vi "TCSPD.VI"() -> ()   [LabVIEW 2018, in "Shared_160.lvlib"]
uses:
  Shared_160.lvlib
  Global_Telescopio.vi
  tele.llb/TCSPD Globals.vi
panel:
  in  "OFF AUX":bool
  in  "EMERGÊNCIA":bool
  in  "Telescópio":bool
  out "Instrumento da Missão":string
  in  "Tabela Proteção":string[][](table)=[["Coude", "281.52", " 11.53", "S", "S", "0.462", "23.1", "23.1"], ["Cassegrain", "281.52", " 11.53", "S", "S", "0.462", "23.1", "23.1"], ["Eucalyptus", "281.52", " 11.53", "S", "S", "0.462", "23.1", "23.1"], ["Cam 1", "281.52", " 11.53", "S", "S", "0.462", "23.1", "23.1"], ["Cam 2", "281.52", " 11.53", "S", "S", "0.462", "23.1", "23.1"], ["Cam IV", "281.52", " 11.53", "S", "S", "0.462", "23.1", "23.1"], ["Polarimetro", "281.52", " 11.53", "S", "S", "0.462", "23.1", "23.1"], ["Fortrap", "281.52", " 11.53", "S", "S", "0.462", "23.1", "23.1"]]
  in  "CorrecaoMin":dbl=0.1
  out "Instrumento":u16(ring) items=["Coude A+", "Coude B+", "ECass+", "Eucalyptus+", "Cam 1+", "Cam 2*", "Cam4 + IV*", "Polarimetro*", "Fortrap*", "Cam1 RF*", "Coude C+", "MUSICOS*", "+Já testado", "* nao config", "cam 1 s/rf", "cam1srf/luca+focali", "Coude A/luca", "ECass/luca", "Cam1+rf+luca", "MUSICOS+Luca", "Camiv+Luca", "Cam2+Luca", "Cam1+rf+luca+Ixon", "Cam1+rf+luca+Ikon", "CoudeTeste", "*cam1srf/luca+focali", "cam1 + esp_focal", "SPARC4"]
  in  "tel_sts1":bool[](array[boolean])=[TRUE, TRUE, TRUE, TRUE, FALSE, FALSE, TRUE]
  out "String 4":string
  out "String 2":string
  out "String 3":string
  out "String":string
  in  "Boolean":bool
  out "Data Socket Test":dbl
  out "URL Temperatura":string
  in  "Reset_uC":bool
  in  "Password":string
  out "error out":errorcluster
  in  "sair":bool
  in  "ENGENHARIA":bool
  in  "SETUP":bool
  in  "Web Server:TCP/IP Access List":string[](array[string])=["c+*", "+observacao.vi"]
  # "TCSPD"
  # "TELESCOPE CONTROL SYSTEM\nPICO DOS DIAS OBSERVATORY"
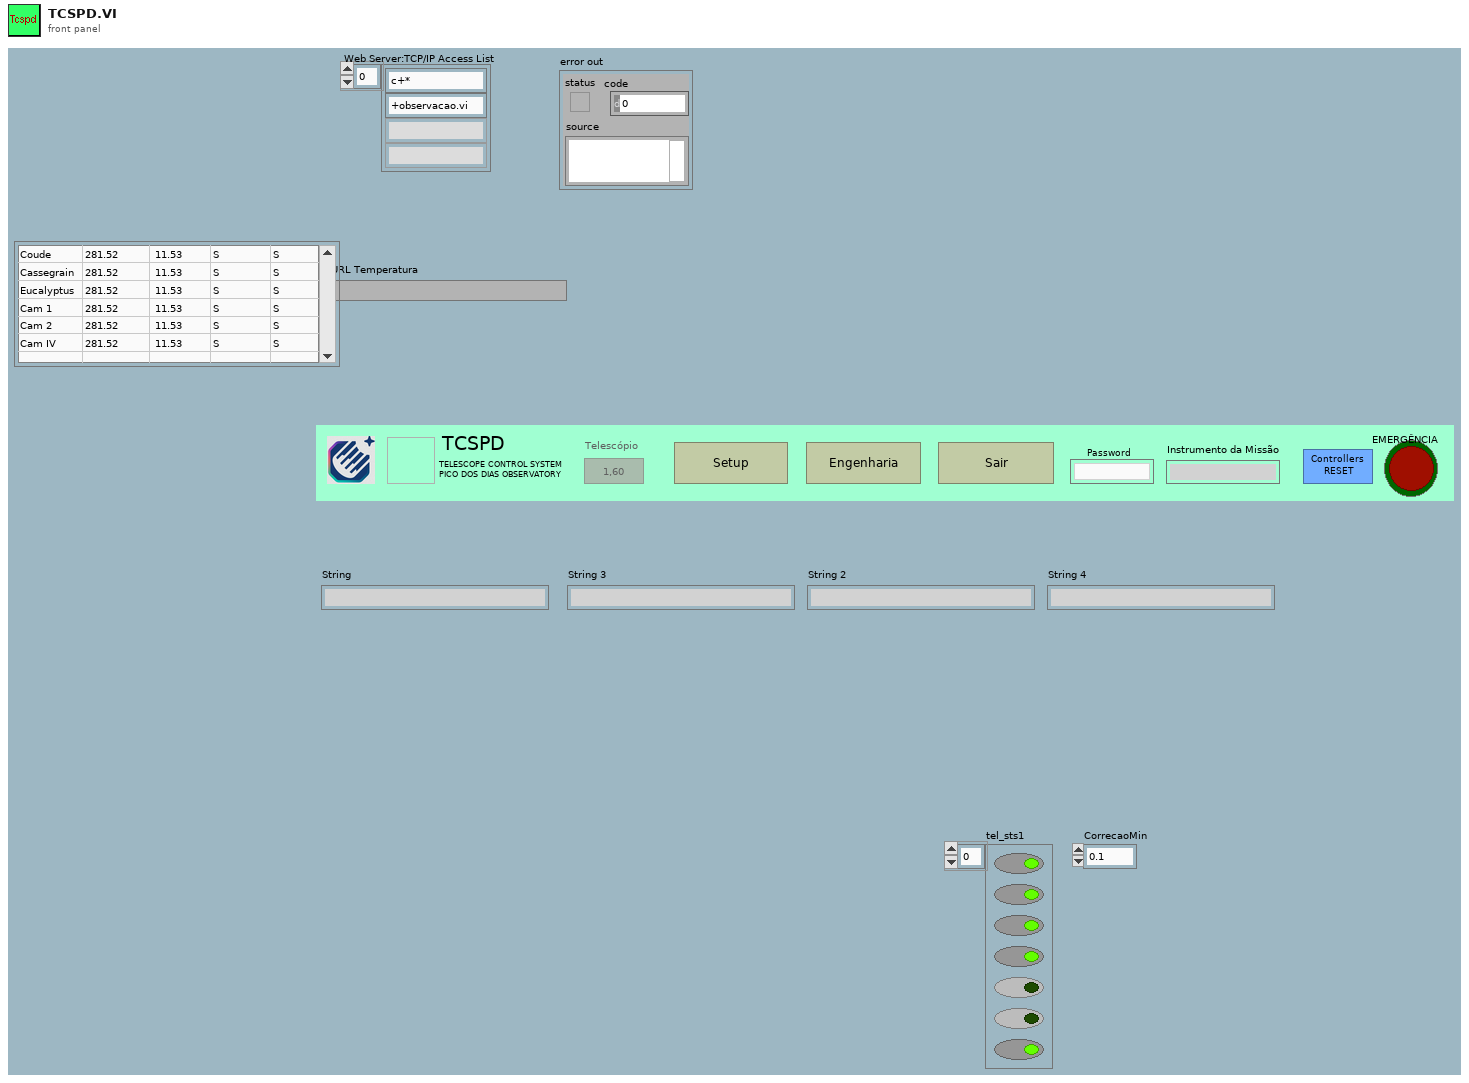
[diagram p1: front panel]
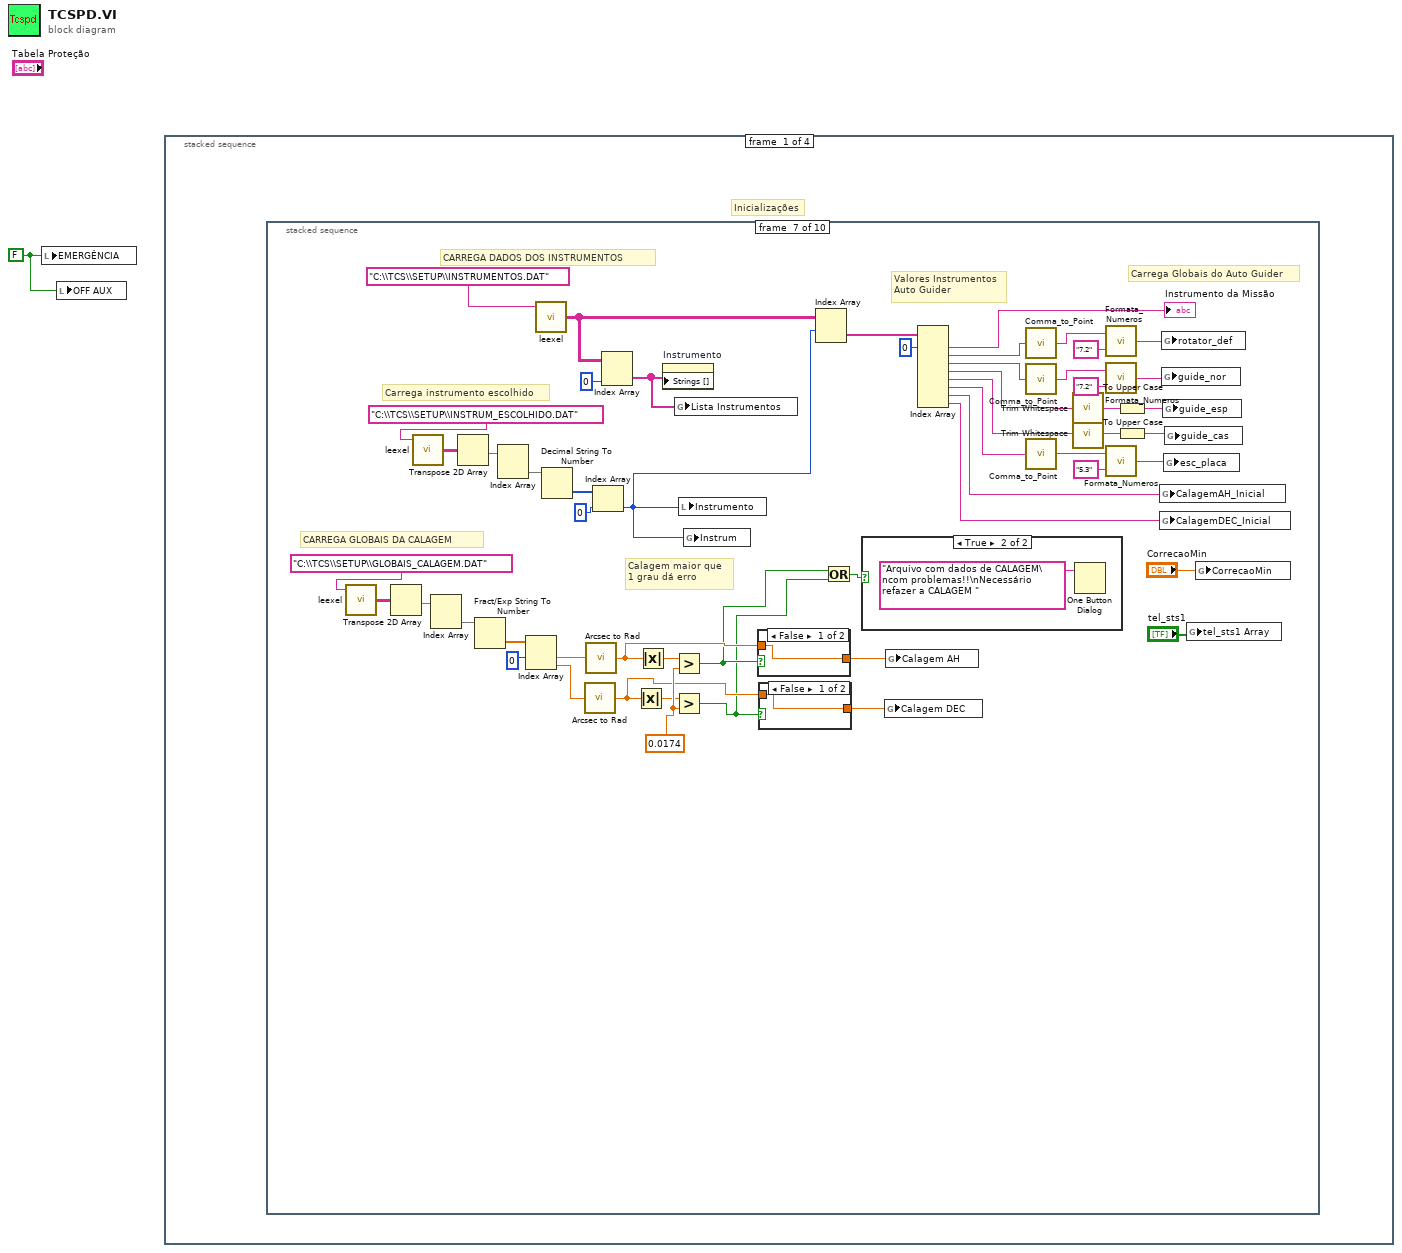
[diagram p0: block diagram]
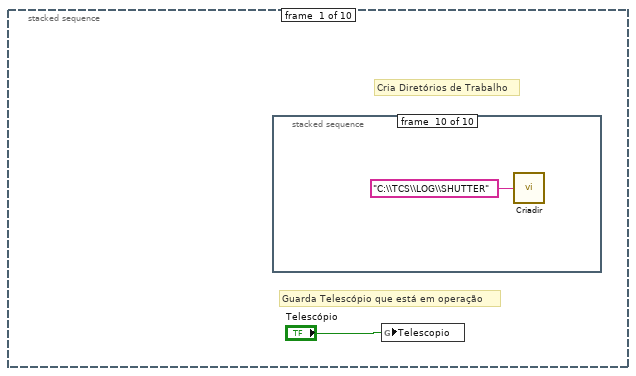
[diagram p2: hidden frame]
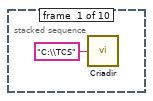
[diagram p3: hidden frame]
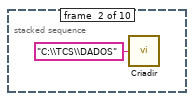
[diagram p4: hidden frame]
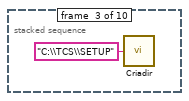
[diagram p5: hidden frame]
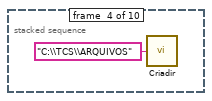
[diagram p6: hidden frame]
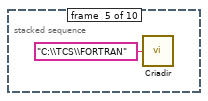
[diagram p7: hidden frame]
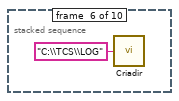
[diagram p8: hidden frame]
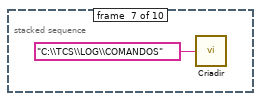
[diagram p9: hidden frame]
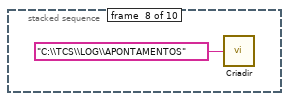
[diagram p10: hidden frame]
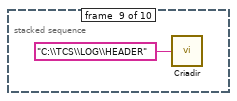
[diagram p11: hidden frame]
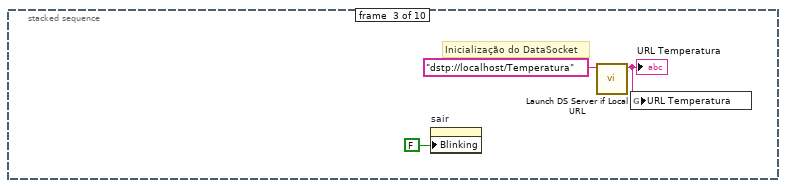
[diagram p13: hidden frame]
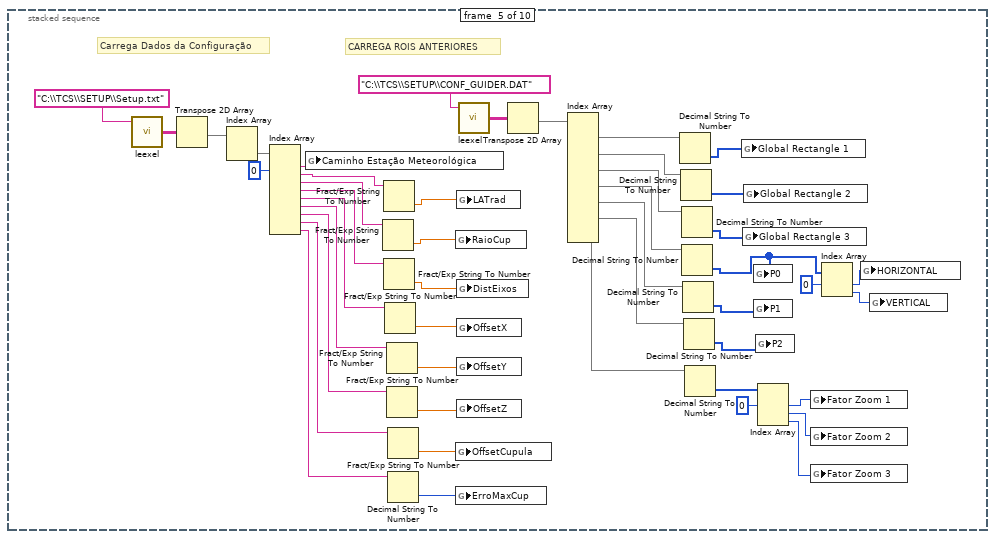
[diagram p15: hidden frame]
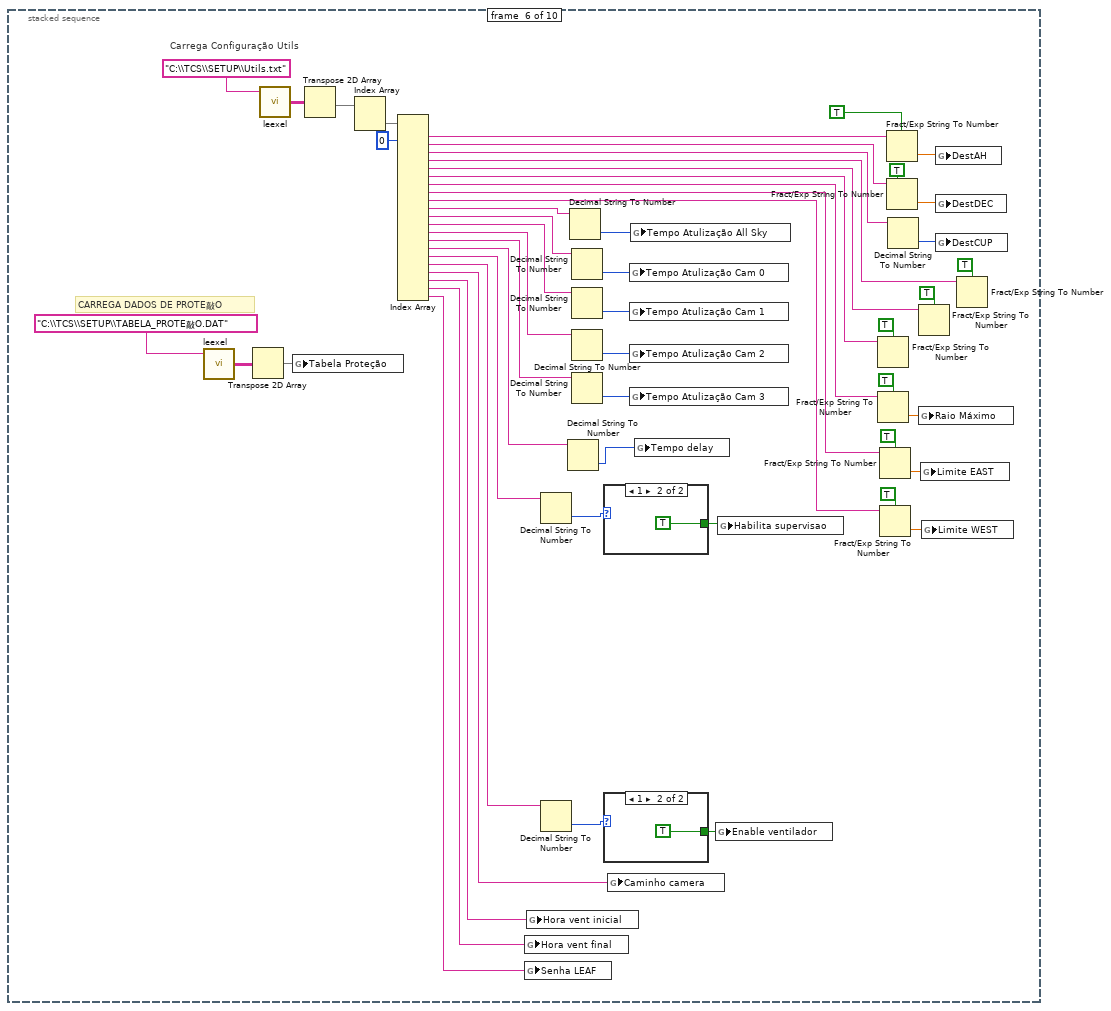
[diagram p16: hidden frame]
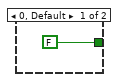
[diagram p17: hidden frame]
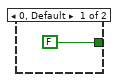
[diagram p18: hidden frame]
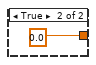
[diagram p20: hidden frame]
diagram:
  w1 = FALSE ("OFF")
  n1 = local write "EMERGÊNCIA"(w1) -> ()
  n2 = local write "OFF AUX"(w1) -> ()
  n3 = stacked-sequence {
    frame #0 {
      # "Inicializações"
      n4 = stacked-sequence {
        frame #0 {
          # "Guarda Telescópio que está em operação"
          # "Cria Diretórios de Trabalho"
          n5 = stacked-sequence {
            frame #0 {
              n6 = call "Criadir.vi"("SOMENTE DIRETORIO"="C:\\TCS") -> ()  [unwired: 2 out]
            }
            frame #1 {
              n7 = call "Criadir.vi"("SOMENTE DIRETORIO"="C:\\TCS\\DADOS") -> ()  [unwired: 2 out]
            }
            frame #2 {
              n8 = call "Criadir.vi"("SOMENTE DIRETORIO"="C:\\TCS\\SETUP") -> ()  [unwired: 2 out]
            }
            frame #3 {
              n9 = call "Criadir.vi"("SOMENTE DIRETORIO"="C:\\TCS\\ARQUIVOS") -> ()  [unwired: 2 out]
            }
            frame #4 {
              n10 = call "Criadir.vi"("SOMENTE DIRETORIO"="C:\\TCS\\FORTRAN") -> ()  [unwired: 2 out]
            }
            frame #5 {
              n11 = call "Criadir.vi"("SOMENTE DIRETORIO"="C:\\TCS\\LOG") -> ()  [unwired: 2 out]
            }
            frame #6 {
              n12 = call "Criadir.vi"("SOMENTE DIRETORIO"="C:\\TCS\\LOG\\COMANDOS") -> ()  [unwired: 2 out]
            }
            frame #7 {
              n13 = call "Criadir.vi"("SOMENTE DIRETORIO"="C:\\TCS\\LOG\\APONTAMENTOS") -> ()  [unwired: 2 out]
            }
            frame #8 {
              n14 = call "Criadir.vi"("SOMENTE DIRETORIO"="C:\\TCS\\LOG\\HEADER") -> ()  [unwired: 2 out]
            }
            frame #9 {
              n15 = call "Criadir.vi"("SOMENTE DIRETORIO"="C:\\TCS\\LOG\\SHUTTER") -> ()  [unwired: 2 out]
            }
          }
          n16 = global write "Global_Telescopio.vi" "Telescopio"("Telescópio") -> ()
        }
        frame #1 {
        }
        frame #2 {
          # "Inicialização do DataSocket"
          n17 = property on="sair" class="Bool"("Blinking"=FALSE) -> ()  [unwired: 2 in, 2 out]
          n18 = call "Launch DS Server if Local URL.vi"("URL"="dstp://localhost/Temperatura") -> ("Duplicate URL"=w14:string)  [unwired: 5 in, 1 out]
          "URL Temperatura" <- w14
          n19 = global write "Global_Telescopio.vi" "URL Temperatura"(w14) -> ()
        }
        frame #3 {
          # "Inicializaqção da placa de imagem Angelo"
        }
        frame #4 {
          # "CARREGA ROIS ANTERIORES"
          # "Carrega Dados da Configuração"
          n20 = call "leexel.vi"("path"="C:\\TCS\\SETUP\\Setup.txt") -> ("array 5"=w60:string[][])  [unwired: 4 in]
          n21 = Transpose 2D Array(2D array=w60) -> (transposed array=w59:string[][])
          n22 = Index Array(array=w59) -> (element=w58:string[])  [unwired: 2 in]
          n23 = Index Array(array=w58, index #1=0 ("index")) -> (element #1=w56:string, element #2=w55:string, element #3=w54:string, element #4=w53:string, element #5=w52:string, element #6=w51:string, element #7=w50:string, element #8=w18:string, element #9=w16:string)  [unwired: 8 in]
          n24 = global write "Global_Telescopio.vi" "Caminho Estação Meteorológica"(w56) -> ()
          n25 = Fract/Exp String To Number(string=w54) -> (number=w48:dbl)  [unwired: 3 in, 1 out]
          n26 = Fract/Exp String To Number(string=w55) -> (number=w49:dbl)  [unwired: 3 in, 1 out]
          n27 = Fract/Exp String To Number(string=w53) -> (number=w47:dbl)  [unwired: 3 in, 1 out]
          n28 = Fract/Exp String To Number(string=w52) -> (number=w46:dbl)  [unwired: 3 in, 1 out]
          n29 = Fract/Exp String To Number(string=w51) -> (number=w45:dbl)  [unwired: 3 in, 1 out]
          n30 = Fract/Exp String To Number(string=w50) -> (number=w44:dbl)  [unwired: 3 in, 1 out]
          n31 = Fract/Exp String To Number(string=w18) -> (number=w19:dbl)  [unwired: 3 in, 1 out]
          n32 = Decimal String To Number(string=w16) -> (number=w17:i32)  [unwired: 2 in, 1 out]
          n33 = global write "Global_Telescopio.vi" "RaioCup"(w48) -> ()
          n34 = global write "Global_Telescopio.vi" "OffsetCupula"(w19) -> ()
          n35 = global write "Global_Telescopio.vi" "ErroMaxCup"(w17) -> ()
          n36 = global write "Global_Telescopio.vi" "LATrad"(w49) -> ()
          n37 = global write "Global_Telescopio.vi" "DistEixos"(w47) -> ()
          n38 = global write "Global_Telescopio.vi" "OffsetX"(w46) -> ()
          n39 = global write "Global_Telescopio.vi" "OffsetY"(w45) -> ()
          n40 = global write "Global_Telescopio.vi" "OffsetZ"(w44) -> ()
          n41 = call "leexel.vi"("path"="C:\\TCS\\SETUP\\CONF_GUIDER.DAT") -> ("array 5"=w42:string[][])  [unwired: 4 in]
          n42 = Transpose 2D Array(2D array=w42) -> (transposed array=w41:string[][])
          n43 = Index Array(array=w41) -> (element #1=w40:string[], element #2=w39:string[], element #3=w38:string[], element #4=w37:string[], element #5=w36:string[], element #6=w35:string[], element #7=w20:string[])  [unwired: 14 in]
          n44 = Decimal String To Number(string=w40) -> (number=w26:i32[])  [unwired: 2 in, 1 out]
          n45 = Decimal String To Number(string=w39) -> (number=w27:i32[])  [unwired: 2 in, 1 out]
          n46 = Decimal String To Number(string=w38) -> (number=w28:i32[])  [unwired: 2 in, 1 out]
          n47 = Decimal String To Number(string=w37) -> (number=w31:i32[])  [unwired: 2 in, 1 out]
          n48 = Decimal String To Number(string=w36) -> (number=w30:i32[])  [unwired: 2 in, 1 out]
          n49 = Decimal String To Number(string=w35) -> (number=w29:i32[])  [unwired: 2 in, 1 out]
          n50 = Decimal String To Number(string=w20) -> (number=w23:i32[])  [unwired: 2 in, 1 out]
          n51 = global write "Global_Telescopio.vi" "Global Rectangle 1"(w26) -> ()
          n52 = global write "Global_Telescopio.vi" "Global Rectangle 3"(w28) -> ()
          n53 = global write "Global_Telescopio.vi" "Global Rectangle 2"(w27) -> ()
          n54 = global write "Global_Telescopio.vi" "P0"(w31) -> ()
          n55 = global write "Global_Telescopio.vi" "P1"(w30) -> ()
          n56 = global write "Global_Telescopio.vi" "P2"(w29) -> ()
          n57 = Index Array(array=w23, index #1=0 ("index")) -> (element #1=w24:i32, element #2=w22:i32, element #3=w21:i32)  [unwired: 2 in]
          n58 = global write "Global_Telescopio.vi" "Fator Zoom 1"(w24) -> ()
          n59 = global write "Global_Telescopio.vi" "Fator Zoom 2"(w22) -> ()
          n60 = global write "Global_Telescopio.vi" "Fator Zoom 3"(w21) -> ()
          n61 = Index Array(array=w31, index #1=0 ("index")) -> (element #1=w33:i32, element #2=w32:i32)  [unwired: 1 in]
          n62 = global write "Global_Telescopio.vi" "HORIZONTAL"(w33) -> ()
          n63 = global write "Global_Telescopio.vi" "VERTICAL"(w32) -> ()
        }
        frame #5 {
          # "CARREGA DADOS DE PROTE敲O"
          # "Carrega Configuração Utils"
          n64 = call "leexel.vi"("path"="C:\\TCS\\SETUP\\TABELA_PROTE敲O.DAT") -> ("array 5"=w92:string[][])  [unwired: 4 in]
          n65 = Transpose 2D Array(2D array=w92) -> (transposed array=w90:string[][])
          n66 = call "leexel.vi"("path"="C:\\TCS\\SETUP\\Utils.txt") -> ("array 5"=w113:string[][])  [unwired: 4 in]
          n67 = global write "Global_Telescopio.vi" "Tabela Proteção"(w90) -> ()
          n68 = Transpose 2D Array(2D array=w113) -> (transposed array=w112:string[][])
          n69 = Index Array(array=w112) -> (element=w111:string[])  [unwired: 2 in]
          n70 = Index Array(array=w111, index #1=0 ("index")) -> (element #1=w109:string, element #2=w108:string, element #3=w107:string, element #4=w98:string, element #5=w97:string, element #6=w96:string, element #7=w93:string, element #8=w77:string, element #9=w76:string, element #10=w80:string, element #11=w81:string, element #12=w82:string, element #13=w83:string, element #14=w84:string, element #15=w71:string, element #16=w70:string, element #17=w66:string, element #18=w65:string, element #19=w64:string, element #20=w63:string, element #21=w62:string)  [unwired: 20 in]
          n71 = global write "Global_Telescopio.vi" "Hora vent final"(w63) -> ()
          n72 = global write "Global_Telescopio.vi" "Senha LEAF"(w62) -> ()
          n73 = global write "Global_Telescopio.vi" "Hora vent inicial"(w64) -> ()
          n74 = Decimal String To Number(string=w70) -> (number=w73:i32)  [unwired: 2 in, 1 out]
          n75 = Decimal String To Number(string=w66) -> (number=w68:i32)  [unwired: 2 in, 1 out]
          n76 = Decimal String To Number(string=w71) -> (number=w69:i32)  [unwired: 2 in, 1 out]
          n77 = Decimal String To Number(string=w80) -> (number=w89:i32)  [unwired: 2 in, 1 out]
          n78 = Decimal String To Number(string=w81) -> (number=w88:i32)  [unwired: 2 in, 1 out]
          n79 = Decimal String To Number(string=w82) -> (number=w87:i32)  [unwired: 2 in, 1 out]
          n80 = Decimal String To Number(string=w83) -> (number=w86:i32)  [unwired: 2 in, 1 out]
          n81 = Decimal String To Number(string=w84) -> (number=w85:i32)  [unwired: 2 in, 1 out]
          n82 = case shown="1" w73 {
            tunnel: [FALSE TRUE] -> w72
            frame 0, Default {
            }
            frame 1 {
            }
          }
          n83 = case shown="1" w68 {
            tunnel: [FALSE TRUE] -> w67
            frame 0, Default {
            }
            frame 1 {
            }
          }
          n84 = global write "Global_Telescopio.vi" "Caminho camera"(w65) -> ()
          n85 = global write "Global_Telescopio.vi" "Tempo Atulização Cam 0"(w88) -> ()
          n86 = global write "Global_Telescopio.vi" "Tempo Atulização Cam 1"(w87) -> ()
          n87 = global write "Global_Telescopio.vi" "Tempo Atulização Cam 2"(w86) -> ()
          n88 = global write "Global_Telescopio.vi" "Tempo Atulização Cam 3"(w85) -> ()
          n89 = global write "Global_Telescopio.vi" "Tempo Atulização All Sky"(w89) -> ()
          n90 = global write "Global_Telescopio.vi" "Tempo delay"(w69) -> ()
          n91 = global write "Global_Telescopio.vi" "Enable ventilador"(w67) -> ()
          n92 = global write "Global_Telescopio.vi" "Habilita supervisao"(w72) -> ()
          n93 = Fract/Exp String To Number(use system decimal point (T)=TRUE, string=w96) -> ()  [unwired: 2 in, 2 out]
          n94 = Fract/Exp String To Number(use system decimal point (T)=TRUE, string=w93) -> (number=w94:dbl)  [unwired: 2 in, 1 out]
          n95 = Fract/Exp String To Number(use system decimal point (T)=TRUE, string=w77) -> (number=w75:dbl)  [unwired: 2 in, 1 out]
          n96 = Fract/Exp String To Number(use system decimal point (T)=TRUE, string=w76) -> (number=w74:dbl)  [unwired: 2 in, 1 out]
          n97 = Fract/Exp String To Number(use system decimal point (T)=TRUE, string=w109) -> (number=w105:dbl)  [unwired: 2 in, 1 out]
          n98 = Fract/Exp String To Number(use system decimal point (T)=TRUE, string=w108) -> (number=w104:dbl)  [unwired: 2 in, 1 out]
          n99 = Decimal String To Number(string=w107) -> (number=w106:i32)  [unwired: 2 in, 1 out]
          n100 = Fract/Exp String To Number(use system decimal point (T)=TRUE, string=w97) -> ()  [unwired: 2 in, 2 out]
          n101 = global write "Global_Telescopio.vi" "Raio Máximo"(w94) -> ()
          n102 = global write "Global_Telescopio.vi" "Limite EAST"(w75) -> ()
          n103 = global write "Global_Telescopio.vi" "Limite WEST"(w74) -> ()
          n104 = global write "Global_Telescopio.vi" "DestAH"(w105) -> ()
          n105 = global write "Global_Telescopio.vi" "DestDEC"(w104) -> ()
          n106 = global write "Global_Telescopio.vi" "DestCUP"(w106) -> ()
          n107 = Fract/Exp String To Number(use system decimal point (T)=TRUE, string=w98) -> ()  [unwired: 2 in, 2 out]
        }
        frame #6 {
          w128 = 0.0174 ("Calagem DEC")
          # "Calagem maior que\n1 grau dá erro"
          # "CARREGA GLOBAIS DA CALAGEM"
          # "Carrega instrumento escolhido"
          # "CARREGA DADOS DOS INSTRUMENTOS"
          # "Carrega Globais do Auto Guider"
          # "Valores Instrumentos\nAuto Guider"
          n108 = call "leexel.vi"("path"="C:\\TCS\\SETUP\\GLOBAIS_CALAGEM.DAT") -> ("array 5"=w156:string[][])  [unwired: 4 in]
          n109 = Transpose 2D Array(2D array=w156) -> (transposed array=w155:string[][])
          n110 = call "leexel.vi"("path"="C:\\TCS\\SETUP\\INSTRUM_ESCOLHIDO.DAT") -> ("array 5"=w149:string[][])  [unwired: 4 in]
          n111 = Index Array(array=w155) -> (element=w157:string[])  [unwired: 2 in]
          n112 = Transpose 2D Array(2D array=w149) -> (transposed array=w150:string[][])
          n113 = Fract/Exp String To Number(string=w157) -> (number=w153:dbl[])  [unwired: 3 in, 1 out]
          n114 = Index Array(array=w150) -> (element=w148:string[])  [unwired: 2 in]
          n115 = Index Array(array=w153, index #1=0 ("index")) -> (element #1=w138:dbl, element #2=w137:dbl)  [unwired: 1 in]
          n116 = call "leexel.vi"("path"="C:\\TCS\\SETUP\\INSTRUMENTOS.DAT") -> ("array 5"=w159:string[][])  [unwired: 4 in]
          n117 = Decimal String To Number(string=w148) -> (number=w152:i32[])  [unwired: 2 in, 1 out]
          n118 = call "Arcsec to Rad.vi"("Arcsec"=w137) -> ("rad"=w122:dbl)
          n119 = call "Arcsec to Rad.vi"("Arcsec"=w138) -> ("rad"=w123:dbl)
          n120 = Index Array(array=w152, index=0) -> (element=w141:i32)
          n121 = Index Array(array=w159, index (col)=0 ("disabled index (col)")) -> (element=w142:string[])  [unwired: 1 in]
          n122 = Absolute Value(x=w122) -> (abs(x)=w127:dbl)
          n123 = Absolute Value(x=w123) -> (abs(x)=w126:dbl)
          n124 = property on="Instrumento" class="Ring (strict)"("Strings []"=w142) -> ()  [unwired: 2 in, 2 out]
          n125 = Greater?(x=w126, y=w128) -> (0:w120:bool)
          n126 = Greater?(x=w127, y=w128) -> (0:w119:bool)
          n127 = global write "Global_Telescopio.vi" "Lista Instrumentos"(w142) -> ()
          n128 = local write "Instrumento"(w141) -> ()
          n129 = global write "Global_Telescopio.vi" "Instrum"(w141) -> ()
          n130 = case shown="False" w120 {
            tunnel: [w176 0.0 ("Calagem DEC")] -> w125
            tunnel: w123 -> [w176 _]
            frame False {
            }
            frame True {
            }
          }
          n131 = case shown="False" w119 {
            tunnel: [w174 0.0 ("Calagem DEC")] -> w124
            tunnel: w122 -> [w174 _]
            frame False {
            }
            frame True {
            }
          }
          n132 = Index Array(array=w159, index (row)=w141) -> (element=w161:string[])  [unwired: 1 in]
          n133 = Or(x=w120, y=w119) -> (x .or. y?=w121:bool)
          n134 = case shown="True" w121 {
            frame False {
            }
            frame True {
              n135 = One Button Dialog(message="Arquivo com dados de CALAGEM\ncom problemas!!\nNecessário refazer a CALAGEM ") -> ()  [unwired: 1 in, 1 out]
            }
          }
          n136 = global write "Global_Telescopio.vi" "Calagem DEC"(w124) -> ()
          n137 = global write "Global_Telescopio.vi" "Calagem AH"(w125) -> ()
          n138 = Index Array(array=w161, index #1=0 ("index")) -> (element #1=→"Instrumento da Missão":string, element #2=w130:string, element #3=w131:string, element #4=w132:string, element #5=w133:string, element #6=w134:string, element #7=w135:string, element #8=w136:string)  [unwired: 7 in]
          n139 = call "Comma_to_Point.vi"("Lat_A"=w130) -> ("Saída"=w144:string)
          n140 = call "Comma_to_Point.vi"("Lat_A"=w131) -> ("Saída"=w143:string)
          n141 = call "Comma_to_Point.vi"("Lat_A"=w134) -> ("Saída"=w140:string)
          n142 = call <vilib>:"Trim Whitespace.vi"("string"=w132) -> ("trimmed string"=w167:string)  [unwired: 1 in]
          n143 = call <vilib>:"Trim Whitespace.vi"("string"=w133) -> ("trimmed string"=w166:string)  [unwired: 1 in]
          n144 = call "Formata_Numeros.vi"("Formato ex-> 7.2"="7.2", "Valor num"=w144) -> ("resulting string"=w169:string)
          n145 = call "Formata_Numeros.vi"("Formato ex-> 7.2"="7.2", "Valor num"=w143) -> ("resulting string"=w168:string)
          n146 = call "Formata_Numeros.vi"("Formato ex-> 7.2"="5.3", "Valor num"=w140) -> ("resulting string"=w165:string)
          n147 = To Upper Case(1:w167) -> (0:w163:string)
          n148 = To Upper Case(1:w166) -> (0:w162:string)
          n149 = global write "Global_Telescopio.vi" "CalagemAH_Inicial"(w135) -> ()
          n150 = global write "Global_Telescopio.vi" "CalagemDEC_Inicial"(w136) -> ()
          n151 = global write "Global_Telescopio.vi" "rotator_def"(w169) -> ()
          n152 = global write "Global_Telescopio.vi" "guide_nor"(w168) -> ()
          n153 = global write "Global_Telescopio.vi" "guide_esp"(w163) -> ()
          n154 = global write "Global_Telescopio.vi" "esc_placa"(w165) -> ()
          n155 = global write "Global_Telescopio.vi" "guide_cas"(w162) -> ()
          n156 = global write "Global_Telescopio.vi" "tel_sts1 Array"("tel_sts1") -> ()
          n157 = global write "Global_Telescopio.vi" "CorrecaoMin"("CorrecaoMin") -> ()
        }
        frame #7 {
          (unwired) "c:\\TCS\\ARQUIVOS\\"
          (unwired) "c:\\inetpub\\wwwroot\\ppc\\"
          # "globais do PDA"
          # "nome do arquivo display de saída"
          # "arquivo modelo para display do Telescopio"
          # "arquivo modelo para display do Foco"
          # "pasta onde estão os arquivos modelo para display"
          # "arquivo modelo para display da Cupula"
          # "pasta onde se encontra o arquivo acima"
          # "arquivo escrito pelo ppc.cgi"
          n158 = global write "TCSPD Globals.vi" "Tela do PDA"("") -> ()
          n159 = global write "TCSPD Globals.vi" "Parâmetros"(string[] [] ("Parâmetros")) -> ()
          n160 = global write "TCSPD Globals.vi" "ppcDspCupula name"("ppcDspCupula.asp") -> ()
          n161 = global write "TCSPD Globals.vi" "ppcDspTelescopio name"("ppcDspTelescopio.asp") -> ()
          n162 = global write "TCSPD Globals.vi" "ppcDspFoco name"("ppcDspFoco.asp") -> ()
          n163 = global write "TCSPD Globals.vi" "ppc name"("ppc.txt") -> ()
          n164 = global write "TCSPD Globals.vi" "ppcDisplay name"("ppcDspMain.asp") -> ()
          n165 = global write "TCSPD Globals.vi" "ppcDsp home"("c:\\TCS\\WEB\\") -> ()
          n166 = global write "TCSPD Globals.vi" "ppc home"("c:\\TCS\\ARQUIVOS\\") -> ()
        }
        frame #8 {
          # "Inicialização das Seriais"
        }
        frame #9 {
          # "PORTA COM6"
          # "INICIALIZA敲O DOS MOTORES DO COUDE (PRISMA, ESPELHO, FENDA,REDE)"
          n167 = flat-sequence {
            frame #0 {
              n168 = call "InstrumentControl.vi"("Input Message"="COUDE PRISMA CARREGAR_CONFIG") -> ()  [unwired: 9 in, 2 out]
              n169 = call "InstrumentControl.vi"("Input Message"="COUDE FENDA CARREGAR_CONFIG") -> ()  [unwired: 9 in, 2 out]
              n170 = call "InstrumentControl.vi"("Input Message"="COUDE ESPELHO CARREGAR_CONFIG") -> ()  [unwired: 9 in, 2 out]
              n171 = call "InstrumentControl.vi"("Input Message"="COUDE SERIAL CARREGAR_CONFIG") -> ()  [unwired: 9 in, 2 out]
              n172 = call "InstrumentControl.vi"("Input Message"="COUDE REDE CARREGAR_CONFIG") -> ()  [unwired: 9 in, 2 out]
            }
            frame #1 {
              n173 = case shown="0, Default" 0 {
                frame 0, Default {
                }
                frame 1 {
                  n174 = call "InstrumentControl.vi"("Input Message"="COUDE FENDA INICIAR") -> ()  [unwired: 9 in, 2 out]
                }
                frame 2 {
                  n175 = call "InstrumentControl.vi"("Input Message"="COUDE ESPELHO INICIAR") -> ()  [unwired: 9 in, 2 out]
                }
                frame 3 {
                  n176 = call "InstrumentControl.vi"("Input Message"="COUDE PRISMA INICIAR") -> ()  [unwired: 9 in, 2 out]
                }
                frame 4 {
                  n177 = call "InstrumentControl.vi"("Input Message"="COUDE REDE INICIAR") -> ()  [unwired: 9 in, 2 out]
                }
                frame 5 {
                  n178 = call "InstrumentControl.vi"("Input Message"="COUDE FENDA INICIAR") -> ()  [unwired: 9 in, 2 out]
                  n179 = call "InstrumentControl.vi"("Input Message"="COUDE ESPELHO INICIAR") -> ()  [unwired: 9 in, 2 out]
                  n180 = call "InstrumentControl.vi"("Input Message"="COUDE PRISMA INICIAR") -> ()  [unwired: 9 in, 2 out]
                  n181 = call "InstrumentControl.vi"("Input Message"="COUDE REDE INICIAR") -> ()  [unwired: 9 in, 2 out]
                }
              }
            }
          }
        }
      }
    }
    frame #1 {
      # "ZeroMQ"
      # "Rotinas Servidas"
      # "O VI  \"Observacao\" (que será acessada  remotamente) deve ser previamente configurada para o servidor, como segue:\n    - Abra a Vi,\n    - Vá em Tools --> Web Publishing tools\n    - No local VI name aperacerá o nome da VI:\n      não Mexer nesse nome\n    - Deixar como Embedded\n    - Deixar com borda\n    - Colocar em branco (limpar) os campos:\n       Document Title\n       Header\n       Footer\n\nDepois disso é possível olhar um Preview da página e salvá-la no disco.\n\nQuando voce salva no disco, é criado um arquivo .htm no diretório:\nC:\\Arquivos de programas\\National Instruments\\LabVIEW 7.1\\www  (Ex:observacao.htm) que será usado pelo servidor como configuração, quando chamado pelo property node APP acima, e poderá ser acessado remotamente.\n\nRepetir esse processo para outros VIs que eventualmente serão acessados remotamente."
      # "Endereço URL para abrir remotamente\n\nhttp://mct/observacao.htm (rede interna)\nhttp://200.131.64.236/observacao.htm"
      n182 = disable-structure shown="Disabled" {
        disable-tunnel: ["Web Server:TCP/IP Access List" _] -> w205
        disable-tunnel: [w254 _] -> w203
        frame Disabled {
          w254 = path "C:/Arquivos de programas/National Instruments/LabVIEW 7.1/www" ("Web Server:Root Directory Path")
          # "VI´s de acesso remoto."
          # "Liga Servidor e \nLista de Acces list"
          n183 = property class="App" props=["Web Server:Root Directory Path", "Web Server:Server Active", "Web Server:TCP/IP Access List", "Web Server:Server Active"]("Web Server:Root Directory Path"=w254, "Web Server:Server Active"=TRUE, "Web Server:TCP/IP Access List"="Web Server:TCP/IP Access List") -> (error out=→"error out":errorcluster)  [unwired: 2 in, 2 out]
        }
        frame Enabled {
        }
      }
      n184 = while {
        tunnel: [FALSE ("Web Server:Server Active")] -> w202
        tunnel: [w220] -> w206
        tunnel: w205 -> [w220]
        tunnel: [w219] -> w204
        tunnel: w203 -> [w219]
        stop <- "sair" stop-if-true
        # "MUDANÇA: 10/12/2010\nIndicador \"Instrumento da Missão\" substituiu o indicador tipo ring \"Instrumento\". Depois de confirmar que o funcionamento está OK, apagar referências a \"Instrumento\""
        # "Perguntar\nao Saulo"
        # "Perguntar\nao Rodrigo"
        n185 = Equal?(x="lnaengen", y="Password") -> (x = y?=w226:bool)
        n186 = case shown="True" "Boolean" {
          frame False {
          }
          frame True {
            n187 = stacked-sequence {
              frame #0 {
                n188 = call "Comando_Enet_1.vi"("String Enviado Canal 0"="AH EIXO CANAL1") -> ("String  Recebido Canal 0"=→"String":string)  [unwired: 3 in, 1 out]
              }
              frame #1 {
                n189 = call "Comando_Enet_2.vi"("String Enviado Canal 0"="AH EIXO CANAL2") -> ("String  Recebido Canal 0"=→"String 2":string)  [unwired: 3 in, 1 out]
              }
              frame #2 {
                n190 = call "Comando_Enet_3.vi"("String Enviado Canal 0"="AH EIXO CANAL3") -> ("String  Recebido Canal 0"=→"String 3":string)  [unwired: 3 in, 1 out]
              }
              frame #3 {
                n191 = call "Comando_Enet_4.vi"("String Enviado Canal 0"="AH EIXO CANAL4") -> ("String  Recebido Canal 0"=→"String 4":string)  [unwired: 3 in, 1 out]
              }
            }
          }
        }
        n192 = And(x="ENGENHARIA", y=w226) -> (x .and. y?=w217:bool)
        n193 = Equal?(x="lnareset", y="Password") -> (x = y?=w224:bool)
        n194 = global read "Global_Telescopio.vi" "Lista Instrumentos"() -> (w212:string[])
        n195 = And(x="Reset_uC", y=w224) -> (x .and. y?=w218:bool)
        n196 = case shown="False" "EMERGÊNCIA" {
          frame False {
            n197 = case shown="True" "OFF AUX" {
              frame False {
              }
              frame True {
                w236 = u16 3 items=["ZERO", "AH", "DEC", "TUBO", "CUP"] ("Controlador")
                n198 = local write "OFF AUX"(FALSE ("OFF AUX")) -> ()
                n199 = call "Monta comando comFilas .vi"("Comando"="DESLIGAR" ("Dispositivo"), "Dispositivo"="EMERGENCIA", "Controlador"=w236) -> ()  [unwired: 3 in, 4 out]
              }
            }
          }
          frame True {
            n200 = local read "OFF AUX"() -> (w239:bool)
            n201 = case shown="False" w239 {
              frame False {
                w241 = u16 3 items=["ZERO", "AH", "DEC", "TUBO", "CUP"] ("Controlador")
                n202 = local write "OFF AUX"(TRUE ("OFF AUX")) -> ()
                n203 = call "Monta comando comFilas .vi"("Comando"="LIGAR" ("Dispositivo"), "Dispositivo"="EMERGENCIA", "Controlador"=w241) -> ()  [unwired: 3 in, 4 out]
              }
              frame True {
              }
            }
          }
        }
        n204 = global read "Global_Telescopio.vi" "Instrum"() -> (w211:u16)
        "Instrumento" <- w211
        n205 = Or(x=w217, y=w218) -> (x .or. y?=w216:bool)
        n206 = case shown="True" w218 {
          selector: w218 -> [_ w245]
          frame False {
          }
          frame True {
            n207 = call "Reset uC.vi"("CUP"=w245) -> ()  [unwired: 4 in]
          }
        }
        n208 = property on="Instrumento" class="Ring (strict)"("Strings []"=w212) -> ()  [unwired: 2 in, 2 out]
        n209 = global read "Global_Telescopio.vi" "Temperatura"() -> (→"Data Socket Test":dbl)
        n210 = Equal?(x="lnasetup", y="Password") -> (x = y?=w225:bool)
        n211 = Index Array(array=w212, index=w211) -> (element=w210:string)
        n212 = And(x="SETUP", y=w225) -> (x .and. y?=w214:bool)
        n213 = Or(x=w214, y=w216) -> (x .or. y?=w215:bool)
        n214 = local write "Instrumento da Missão"(w210) -> ()
        n215 = case shown="True" w215 {
          frame False {
          }
          frame True {
            n216 = local write "Password"("") -> ()
          }
        }
        n217 = case shown="True" w214 {
          frame False {
          }
          frame True {
            n218 = call "Setup.vi"() -> ()  [unwired: 1 in]
          }
        }
        n219 = Wait Until Next ms Multiple(millisecond multiple=u32 200) -> ()  [unwired: 1 out]
        n220 = global write "Global_Telescopio.vi" "stop"("sair") -> ()
        n221 = property on="sair" class="Bool"("Blinking"="sair") -> ()  [unwired: 2 in, 2 out]
      }
      n222 = call "Data_Socket.vi"() -> ()  [unwired: 1 in]
      n223 = call "QBridge 0MQ focuser.vi"() -> ()  [unwired: 11 in, 1 out]
      n224 = call "QBridge 0MQ weather.vi"() -> ()  [unwired: 11 in, 1 out]
      n225 = call "StatusPub0MQ.vi"() -> ()  [unwired: 11 in, 1 out]
      n226 = call "observacao.vi"() -> ()  [unwired: 1 in]
      n227 = call "Bridge serial.vi"() -> ()  [unwired: 12 in]
      n228 = disable-structure shown="Disabled" {
        disable-tunnel: w206 -> [w260 _]
        disable-tunnel: w204 -> [w259 _]
        disable-tunnel: w202 -> [w258 _]
        frame Disabled {
          # "Desliga Servidor e Lista de Acces list"
          n229 = property class="App" props=["Web Server:Root Directory Path", "Web Server:Server Active", "Web Server:TCP/IP Access List", "Web Server:Server Active"]("Web Server:Root Directory Path"=w259, "Web Server:Server Active"=w258, "Web Server:TCP/IP Access List"=w260) -> ()  [unwired: 2 in, 3 out]
        }
        frame Enabled {
        }
      }
      n230 = Not(x=w202) -> (.not. x?=w207:bool)
      n231 = case shown="True" FALSE {
        tunnel: w207 -> [_ w261]
        frame False {
        }
        frame True {
          n232 = Quit LabVIEW(quit? (T)=w261) -> ()
        }
      }
    }
    frame #2 {
      # "Escreve o log da versão do programa"
      # "MUDANÇA: 20/05/2011\nIncluído RESET dos controladores, exceto\no da cúpula."
      # "RESET DOS CONTROLADORES"
      # "Salva as Globais Calagem"
      n233 = global read "Global_Telescopio.vi" "Calagem AH"() -> (w266:dbl)
      n234 = global read "Global_Telescopio.vi" "Calagem DEC"() -> (w265:dbl)
      n235 = call "Reset uC.vi"() -> ()  [unwired: 5 in]
      n236 = call "Rad to Arcsec.vi"("Radiano"=w266) -> ("Arcsec"=w263:dbl)
      n237 = call "Rad to Arcsec.vi"("Radiano"=w265) -> ("Arcsec"=w264:dbl)
      n238 = Build Array(w263, w264) -> (w273:dbl[])
      n239 = Number To Fractional String(number=w273, precision (6)=i16 8) -> (F-format string=w274:string[])  [unwired: 2 in]
      n240 = Build Array(w274) -> (w268:string[][])
      n241 = String To Path(string="C:\\TCS\\SETUP\\GLOBAIS_CALAGEM.DAT") -> (path=w269:path)
      n242 = Transpose 2D Array(2D array=w268) -> (transposed array=w267:string[][])
      n243 = Delete(path (use dialog)=w269) -> (deleted path=w270:path)  [unwired: 4 in, 2 out]
      n244 = Path To String(path=w270) -> (string=w271:string)
      n245 = call "salvaexel.vi"("appended array"=w267, "file name p/ exell"=w271) -> ()  [unwired: 1 in, 1 out]
      n246 = call "Salva_systems_messages.vi"("Mensagem"="Versão atual TCSPD: 08-06-2022 - Finalizada" ("message")) -> ()  [unwired: 5 in]
    }
    frame #3 {
      n247 = Quit LabVIEW(quit? (T)=TRUE) -> ()
    }
  }
